vi "LDA_Get_4_points.vi"(0 "Beam Data":T1={"Vg1 (Green 1 dir. vect.)"=[0.0, 0.0, 0.0], "Vg2  (Green 2 dir. vect.)"=[0.0, 0.0, 0.0], "Vb1 (Blue 1 dir. vect.)"=[0.0, 0.0, 0.0], "Vb2 (Blue 1 dir. vect.)"=[0.0, 0.0, 0.0], "Porb (Orb XYZ posn. forced coplanar)"=[0.0, 0.0, 0.0], "Porb (Orb XYZ posn. - allow skew)"=[0.0, 0.0, 0.0], "Orb posn. uncertainty, +/- dx, dy, dz"=[0.0, 0.0, 0.0], "Vp (Actual Probe dir. vect)"=[0.0, 0.0, 0.0], "Yaw (deg)"=0.0, "Pitch (deg)"=0.0, "In-Plane Roll (deg)"=0.0, "Beam Half Angle (deg)"=0.0, "B1 Close P11"=[0.0, 0.0, 0.0], "B1 Far P12"=[0.0, 0.0, 0.0], "B2 Close P22"=[0.0, 0.0, 0.0], "B2 Far P21"=[0.0, 0.0, 0.0], "Projected Roll (deg)"=0.0, "Green Velocity Vector"=[0.0, 0.0, 0.0], "Blue Velocity Vector"=[0.0, 0.0, 0.0], "Probe is facing...."="-", "Calculation Method"=""} {"Vp (Actual Probe dir. vect)" format="%#_6f"; "Vg2  (Green 2 dir. vect.)" format="%#_6f"; "Vg1 (Green 1 dir. vect.)" format="%#_6f"}, 1 "L, Probe-Normal Distance":dbl=500.0 format="%#.3g") -> (2 "Pg1":dbl[](array[numeric]) format="%#.3g", 3 "Pg2":dbl[](array[numeric]) format="%#.3g", 4 "Pb1":dbl[](array[numeric]) format="%#.3g", 5 "Pb2":dbl[](array[numeric]) format="%#.3g")   [LabVIEW 2011]
uses:
  Controls/LDA_Beam_Cluster.ctl
  <vilib>/Analysis/baseanly.llb/Real Dot Product.vi
  <vilib>/Analysis/NI_AALBase.lvlib
panel:
  # "Probe positions to achieve beam-orb marriage"
  # "IMPORTANT NOTE:\n\nAll direction vectors MUST be imported normalised!!\n(This is carried out in the vi \"LDA_math_check.vi\")\n\nVp, Vgn and Vbn must be altered as a group, so if probe\nis rotated, then such a transform has to be applied to \nall the direction vectors as well\n(use vi \"Vector3_Rotate\"."
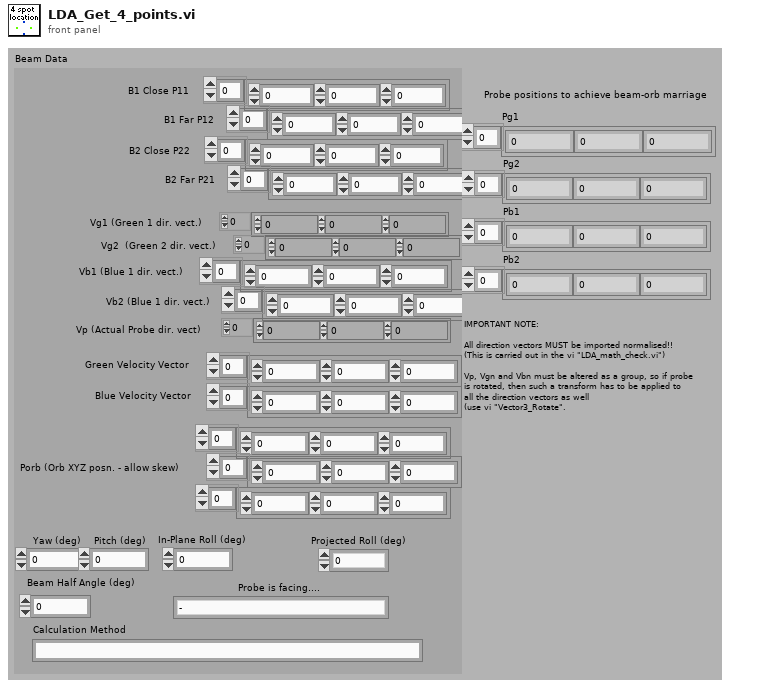
[diagram p1: front panel]
types:
  T1 = typedef "LDA_Beam_Cluster.ctl" = cluster{"Vg1 (Green 1 dir. vect.)":dbl[], "Vg2  (Green 2 dir. vect.)":dbl[], "Vb1 (Blue 1 dir. vect.)":dbl[], "Vb2 (Blue 1 dir. vect.)":dbl[], "Porb (Orb XYZ posn. forced coplanar)":dbl[], "Porb (Orb XYZ posn. - allow skew)":dbl[], "Orb posn. uncertainty, +/- dx, dy, dz":dbl[], "Vp (Actual Probe dir. vect)":dbl[], "Yaw (deg)":dbl, "Pitch (deg)":dbl, "In-Plane Roll (deg)":dbl, "Beam Half Angle (deg)":dbl, "B1 Close P11":dbl[], "B1 Far P12":dbl[], "B2 Close P22":dbl[], "B2 Far P21":dbl[], "Projected Roll (deg)":dbl, "Green Velocity Vector":dbl[], "Blue Velocity Vector":dbl[], "Probe is facing....":string, "Calculation Method":string}
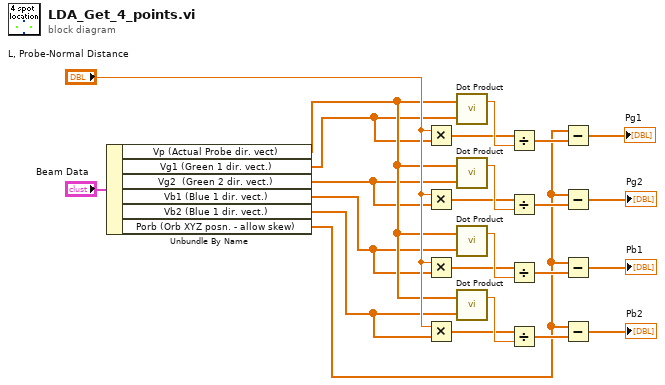
[diagram p0: block diagram]
diagram:
  n1 = Unbundle By Name("Beam Data") -> ("Vp (Actual Probe dir. vect)"=w7:dbl[], "Vg1 (Green 1 dir. vect.)"=w6:dbl[], "Vg2  (Green 2 dir. vect.)"=w5:dbl[], "Vb1 (Blue 1 dir. vect.)"=w4:dbl[], "Vb2 (Blue 1 dir. vect.)"=w3:dbl[], "Porb (Orb XYZ posn. - allow skew)"=w2:dbl[])
  n2 = Multiply(x="L, Probe-Normal Distance", y=w6) -> (x*y=w22:dbl[])
  n3 = Multiply(x="L, Probe-Normal Distance", y=w5) -> (x*y=w20:dbl[])
  n4 = Multiply(x="L, Probe-Normal Distance", y=w4) -> (x*y=w13:dbl[])
  n5 = Multiply(x="L, Probe-Normal Distance", y=w3) -> (x*y=w12:dbl[])
  n6 = call-poly <vilib>:"Dot Product.vi"("Y Vector"=w6, "X Vector"=w7) -> ("X * Y"=w24:dbl)  [unwired: 1 out]
  n7 = call-poly <vilib>:"Dot Product.vi"("Y Vector"=w5, "X Vector"=w7) -> ("X * Y"=w21:dbl)  [unwired: 1 out]
  n8 = call-poly <vilib>:"Dot Product.vi"("Y Vector"=w4, "X Vector"=w7) -> ("X * Y"=w17:dbl)  [unwired: 1 out]
  n9 = call-poly <vilib>:"Dot Product.vi"("Y Vector"=w3, "X Vector"=w7) -> ("X * Y"=w16:dbl)  [unwired: 1 out]
  n10 = Divide(x=w22, y=w24) -> (x/y=w23:dbl[])
  n11 = Divide(x=w20, y=w21) -> (x/y=w19:dbl[])
  n12 = Divide(x=w13, y=w17) -> (x/y=w14:dbl[])
  n13 = Divide(x=w12, y=w16) -> (x/y=w15:dbl[])
  n14 = Subtract(x=w2, y=w23) -> (x-y=→"Pg1":dbl[])
  n15 = Subtract(x=w2, y=w19) -> (x-y=→"Pg2":dbl[])
  n16 = Subtract(x=w2, y=w14) -> (x-y=→"Pb1":dbl[])
  n17 = Subtract(x=w2, y=w15) -> (x-y=→"Pb2":dbl[])
